vi "XML Namespaces.vi"(10 "namespaces to use (empty = all)":string[](array[string]), 11 "String in":string) -> (3 "String out":string)   [LabVIEW 2012]
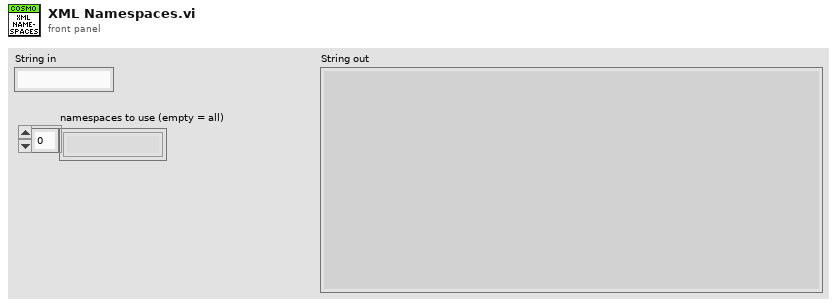
[diagram p1: front panel]
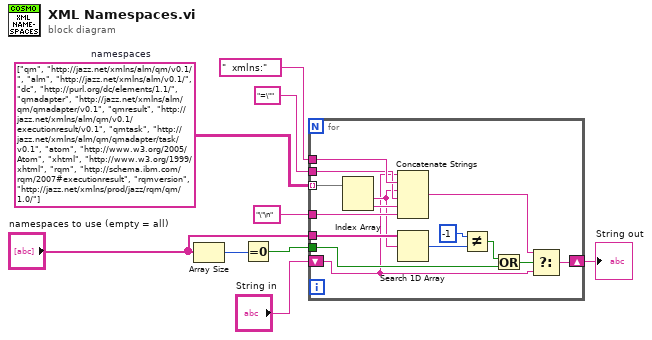
[diagram p0: block diagram]
diagram:
  w4 = string[][] [["qm", "http://jazz.net/xmlns/alm/qm/v0.1/"], ["alm", "http://jazz.net/xmlns/alm/v0.1/"], ["dc", "http://purl.org/dc/elements/1.1/"], ["qmadapter", "http://jazz.net/xmlns/alm/qm/qmadapter/v0.1"], ["qmresult", "http://jazz.net/xmlns/alm/qm/v0.1/executionresult/v0.1"], ["qmtask", "http://jazz.net/xmlns/alm/qm/qmadapter/task/v0.1"], ["atom", "http://www.w3.org/2005/Atom"], ["xhtml", "http://www.w3.org/1999/xhtml"], ["rqm", "http://schema.ibm.com/rqm/2007#executionresult"], ["rqmversion", "http://jazz.net/xmlns/prod/jazz/rqm/qm/1.0/"]]  # namespaces
  n1 = Array Size(array="namespaces to use (empty = all)") -> (size(s)=w2:i32)
  n2 = Equal To 0?(x=w2) -> (x = 0?=w1:bool)
  n3 = for {
    tunnel: w4 -> [w23] mode=indexing
    shift-right: [w15] -> w8
    shift-left: "String in" -> [w11]
    tunnel: "  xmlns:" -> [w24]
    tunnel: "=\"" -> [w22]
    tunnel: "\"\n" -> [w20]
    tunnel: "namespaces to use (empty = all)" -> [w19]
    tunnel: w1 -> [w13]
    n4 = Index Array(array=w23) -> (element #1=w18:string, element #2=w21:string)  [unwired: 2 in]
    n5 = Concatenate Strings(w11, w24, w18, w22, w21, w20) -> (w12:string)
    n6 = Search 1D Array(1D array=w19, element=w18) -> (index of element=w17:i32)  [unwired: 1 in]
    n7 = Not Equal?(x=-1, y=w17) -> (x != y?=w10:bool)
    n8 = Or(x=w10, y=w13) -> (x .or. y?=w14:bool)
    n9 = Select(t=w12, s=w14, f=w11) -> (s? t:f=w15:string)
  }
  "String out" <- w8
